vi "Move Z Raster + Scan.vi"(0 "Reference In":refnum<class "_Controller.lvclass">, 1 "VISA resource name":refnum<visa-resource-name>, 2 "Source (0: Channel 1)":u16(ring) items=["Channel 1", "Channel 2", "Channel 3", "Channel 4", "Memory 1", "Memory 2", "Memory 3", "Memory 4", "Function 1", "Function 2", "Function 3", "Function 4", "Function 5", "Function 6", "Function 7", "Function 8"], 3 "Z Number of Steps":string="0", 4 "Initial Direction":bool=TRUE, 5 "Error In":errorcluster) -> (14 "Reference Out":refnum<class "_Controller.lvclass">, 16 "For Loop Count":i32, 17 "A-Scan":waveform(dbl)[](graph), 19 "Error Out":errorcluster)   [LabVIEW 2020]
doc: "This incorporates both the motion of the machine as well as the reading from the oscilloscope in the Z direction. It automates the process of moving along the entire length of the Z desired length, stopping to scan at regular intervals and finally triggering the osciloscope at each scanning point.\n\nArgs:\n\nReference In: Incoming communication (reference) between LabView and the scanning rig controller\nError In: Checks for any errors with the incoming communication (reference)\nVISA Resource Name: Specifies the model of osciloscope being used \nSource (Channel): Specificies the channel that is being triggered for a reading\nZ Number of Steps: Number of steps to cover the entire Z length\nInitial Direction: Direction to move in the Z direction\n\nReturns:\n\nReference Out: Output communnication (reference) between LabView and controller\nError Out: Checks for any error with output communication (reference)\nFor Loop Count: Live indicator of which loop the scan is on which is used in indexing the array for C-scans\nA-Scan: A-scan in the form of a waveform, note it is within a for loop so outputs multiple A-scan's in this VI alone"
uses:
  <instrlib>/Arcus Ethernet Driver 1.0.0/ArcusEthernetComm/classes/Controller/_Controller.lvclass
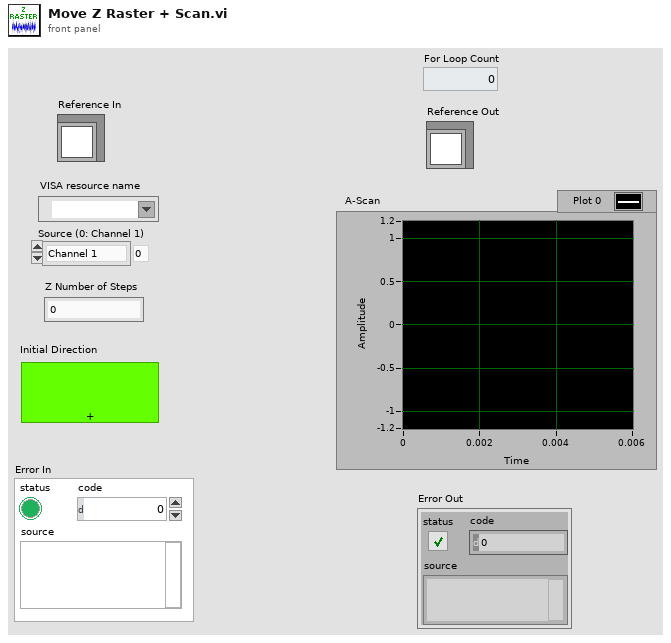
[diagram p1: front panel]
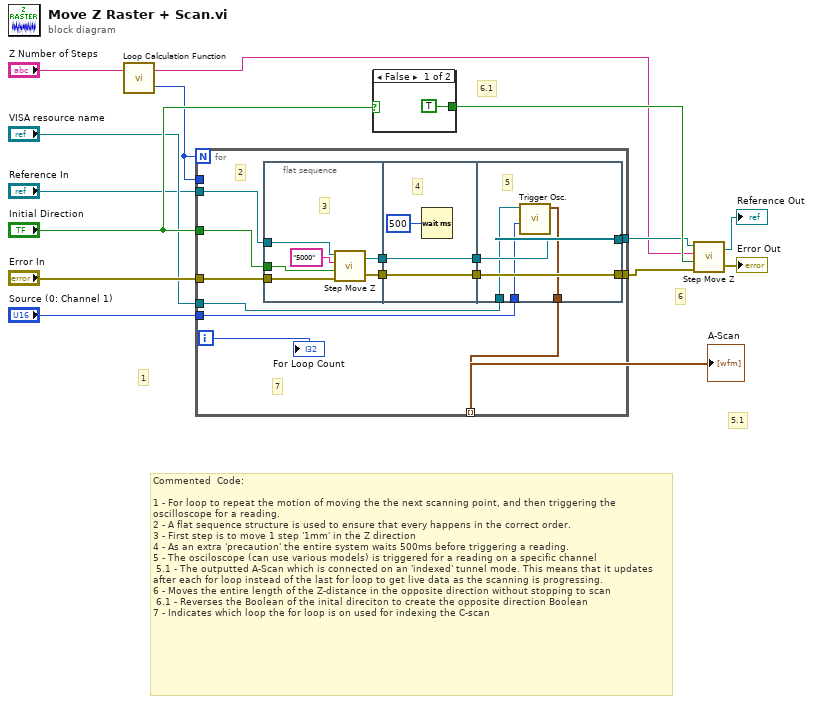
[diagram p0: block diagram]
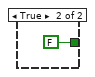
[diagram p2: hidden frame]
diagram:
  # "6.1"
  # "6"
  # "5.1"
  # "1"
  # "Commented  Code: \n\n1 - For loop to repeat the motion of moving the the next scanning point, and then triggering the oscilloscope for a reading.\n2 - A flat sequence structure is used to ensure that every happens in the correct order.\n3 - First step is to move 1 step '1mm' in the Z direction\n4 - As an extra 'precaution' the entire system waits 500ms before triggering a reading.\n5 - The osciloscope (can use various models) is triggered for a reading on a specific channel\n 5.1 - The outputted A-Scan which is connected on an 'indexed' tunnel mode. This means that it updates after each for loop instead of the last for loop to get live data as the scanning is progressing. \n6 - Moves the entire length of the Z-distance in the opposite direction without stopping to scan\n 6.1 - Reverses the Boolean of the inital direciton to create the opposite direction Boolean\n7 - Indicates which loop the for loop is on used for indexing the C-scan"
  n1 = call "Loop Calculation Function.vi"("Number of Steps"="Z Number of Steps") -> ("No. of Scan Points"=w7:i32)  [unwired: 1 in, 1 out]
  n2 = for {
    N: w7 -> [_]
    tunnel: [w26] -> w3
    tunnel: "Initial Direction" -> [w24]
    tunnel: [w25] -> w2
    tunnel: "Reference In" -> [w23]
    tunnel: "Error In" -> [w22]
    tunnel: "VISA resource name" -> [w21]
    tunnel: w7 -> [_]
    tunnel: "Source (0: Channel 1)" -> [w20]
    tunnel: [w19] -> w4 mode=indexing
    i -> [w18]
    # "7"
    # "2"
    n3 = flat-sequence {
      tunnel: w24 -> [w29]
      tunnel: w23 -> [w28]
      tunnel: w22 -> [w27]
      tunnel: [w31] -> w17
      tunnel: [w30] -> w15
      tunnel: w17 -> [w35]
      tunnel: [w35] -> w16
      tunnel: w15 -> [w34]
      tunnel: [w34] -> w14
      tunnel: [w39] -> w25
      tunnel: [w40] -> w26
      tunnel: w16 -> [w40]
      tunnel: w14 -> [w39]
      tunnel: w21 -> [w38]
      tunnel: w20 -> [w37]
      tunnel: [w36] -> w19
      frame #0 {
        # "3"
        n4 = call "Step Move Z.vi"("Error In"=w27, "Direction"=w29, "No. of Z Steps"="5000" ("X Steps"), "Reference In"=w28) -> ("Error Out"=w30:errorcluster, "Reference Out"=w31:refnum<class "_Controller.lvclass">)
      }
      frame #1 {
        # "4"
        n5 = Wait (ms)(milliseconds to wait=u32 500) -> ()  [unwired: 1 out]
      }
      frame #2 {
        # "5"
        n6 = call "Trigger Osc..vi"("Source (0: Channel 1)"=w37, "VISA resource name"=w38) -> ("Waveform Data"=w36:waveform(dbl))  [unwired: 9 in]
      }
    }
    "For Loop Count" <- w18
  }
  "A-Scan" <- w4
  n7 = case shown="False" "Initial Direction" {
    tunnel: [TRUE FALSE] -> w12
    frame False {
    }
    frame True {
    }
  }
  n8 = call "Step Move Z.vi"("Error In"=w2, "Direction"=w12, "No. of Z Steps"="Z Number of Steps", "Reference In"=w3) -> ("Error Out"=→"Error Out":errorcluster, "Reference Out"=→"Reference Out":refnum<class "_Controller.lvclass">)
